vi "Measurement_trial.vi"(0 "I offset":dbl, 2 "input cluster":T1) -> (3 "VR frequency":dbl, 4 "VL frequency":dbl, 5 "PLL output":cluster{dbl, dbl, dbl, dbl}, 6 "RMS values":dbl[](array[numeric]), 7 "Active Power":dbl, 8 "Total power values":dbl[](array[numeric]))   [LabVIEW 2016]
uses:
  <vilib>/measure/matone.llb/Extract Single Tone Information 1 Chan.vi
  <vilib>/measure/NI_MAPro.lvlib
panel:
  in  "dt":dbl=0.000482253 format="%#_13g"
  in  "Numeric":i32=100
  out "I RMS":dbl
  out "VR RMS":dbl
  out "VL RMS":dbl
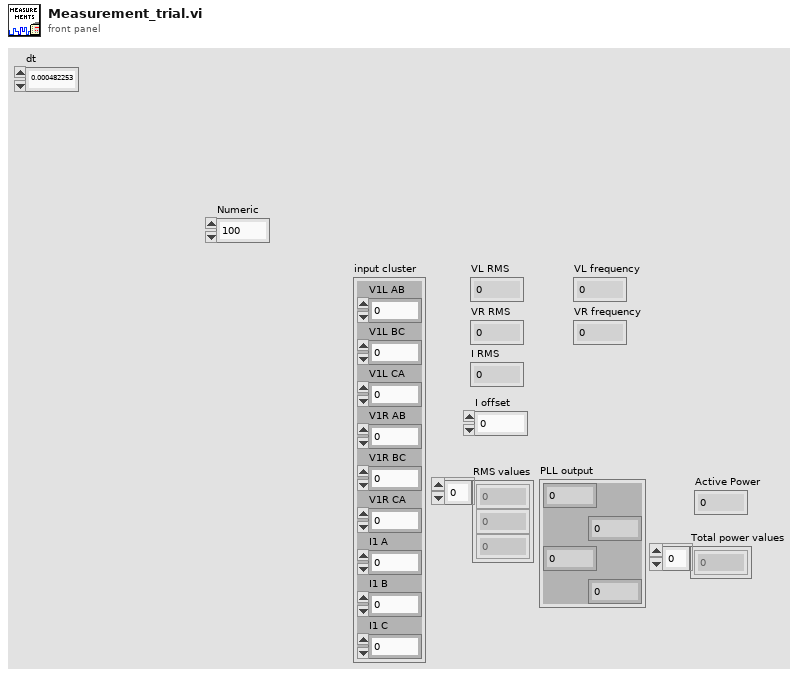
[diagram p1: front panel]
types:
  T1 = cluster{"V1L AB":fxp<+/-,53,11>, "V1L BC":fxp<+/-,53,11>, "V1L CA":fxp<+/-,53,11>, "V1R AB":fxp<+/-,53,11>, "V1R BC":fxp<+/-,53,11>, "V1R CA":fxp<+/-,53,11>, "I1 A":fxp<+/-,53,11>, "I1 B":fxp<+/-,53,11>, "I1 C":fxp<+/-,53,11>}
  T2 = cluster{"V1L AB":fxp<+/-,53,11>, "V1L BC":fxp<+/-,53,11>, "V1L CA":fxp<+/-,53,11>}
  T3 = cluster{"V1R AB":fxp<+/-,53,11>, "V1R BC":fxp<+/-,53,11>, "V1R CA":fxp<+/-,53,11>}
  T4 = cluster{"I1 A":fxp<+/-,53,11>, "I1 B":fxp<+/-,53,11>, "I1 C":fxp<+/-,53,11>}
  T5 = cluster{"t":dbl, "detected phase (deg)":dbl, "detected frequency":dbl, "detected phase (deg)":dbl}
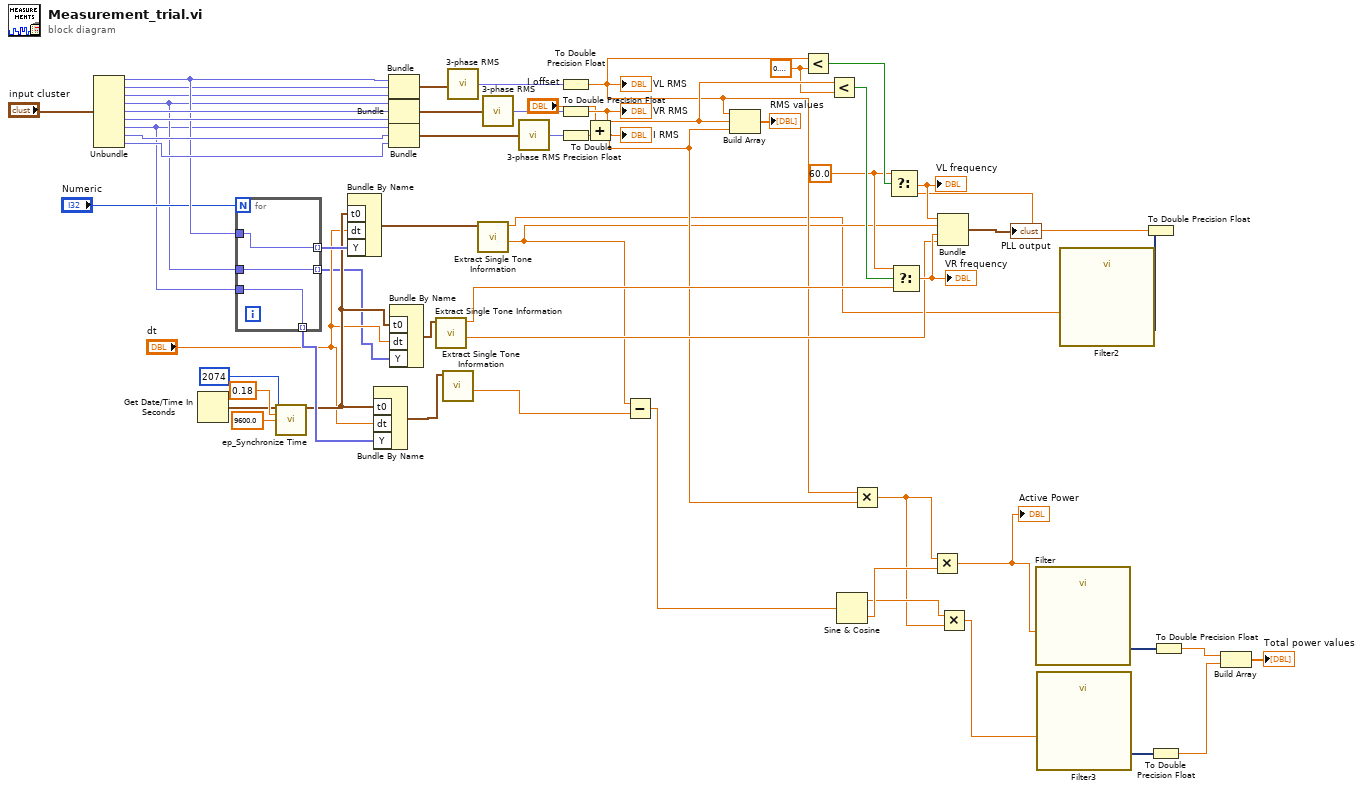
[diagram p0: block diagram]
diagram:
  w48 = 60.0 ("t")
  w51 = 0.30000001192092896 ("y")
  n1 = Unbundle("input cluster") -> ("V1L AB"=w34:fxp<+/-,53,11>, "V1L BC"=w15:fxp<+/-,53,11>, "V1L CA"=w14:fxp<+/-,53,11>, "V1R AB"=w10:fxp<+/-,53,11>, "V1R BC"=w36:fxp<+/-,53,11>, "V1R CA"=w35:fxp<+/-,53,11>, "I1 A"=w9:fxp<+/-,53,11>, "I1 B"=w45:fxp<+/-,53,11>, "I1 C"=w44:fxp<+/-,53,11>)
  n2 = Get Date/Time In Seconds() -> (seconds since 1Jan1904=w28:timestamp)
  n3 = for {
    N: "Numeric" -> [_]
    tunnel: w34 -> [w63]
    tunnel: w10 -> [w62]
    tunnel: [w63] -> w32 mode=indexing
    tunnel: [w62] -> w5 mode=indexing
    tunnel: w9 -> [w61]
    tunnel: [w61] -> w23 mode=indexing
  }
  n4 = call <vilib>:"ep_Synchronize Time.vi"("RT controler time in"=w28, "maximum time difference (sec)"=0.18, "sampling rate (Hz)"=9600.0, "basic calc. interval (samples)"=2074) -> ("RT controler time out"=w7:timestamp)  [unwired: 11 in]
  n5 = Bundle By Name("t0"=w7, "dt"="dt", "Y"=w32) -> (w8:waveform(dbl))  [unwired: 1 in]
  n6 = Bundle By Name("t0"=w7, "dt"="dt", "Y"=w23) -> (w13:waveform(dbl))  [unwired: 1 in]
  n7 = Bundle("V1L AB"=w34, "V1L BC"=w15, "V1L CA"=w14) -> (w59:T2)  [unwired: 1 in]
  n8 = Bundle("V1R AB"=w10, "V1R BC"=w36, "V1R CA"=w35) -> (w58:T3)  [unwired: 1 in]
  n9 = Bundle("I1 A"=w9, "I1 B"=w45, "I1 C"=w44) -> (w57:T4)  [unwired: 1 in]
  n10 = Bundle By Name("t0"=w7, "dt"="dt", "Y"=w5) -> (w4:waveform(dbl))  [unwired: 1 in]
  n11 = call-poly <vilib>:"Extract Single Tone Information.vi"("time signal in"=w4) -> ("detected phase (deg)"=w26:dbl, "detected frequency"=w27:dbl)  [unwired: 5 in, 4 out]
  n12 = call-poly <vilib>:"Extract Single Tone Information.vi"("time signal in"=w13) -> ("detected phase (deg)"=w21:dbl)  [unwired: 5 in, 5 out]
  n13 = call "3-phase RMS.vi"("Vabc"=w59) -> ("RMS"=w55:fxp<+,55,5>)  [unwired: 4 in]
  n14 = call-poly <vilib>:"Extract Single Tone Information.vi"("time signal in"=w8) -> ("detected phase (deg)"=w22:dbl, "detected frequency"=w3:dbl)  [unwired: 5 in, 4 out]
  n15 = call "3-phase RMS.vi"("Vabc"=w58) -> ("RMS"=w54:fxp<+,55,5>)  [unwired: 4 in]
  n16 = call "3-phase RMS.vi"("Vabc"=w57) -> ("RMS"=w56:fxp<+,55,5>)  [unwired: 4 in]
  n17 = To Double Precision Float(number=w55) -> (double precision float=w25:dbl)
  "VL RMS" <- w25
  n18 = To Double Precision Float(number=w54) -> (double precision float=w53:dbl)
  "VR RMS" <- w53
  n19 = To Double Precision Float(number=w56) -> (double precision float=w52:dbl)
  n20 = Add(x="I offset", y=w52) -> (x+y=w24:dbl)
  "I RMS" <- w24
  n21 = Subtract(x=w22, y=w21) -> (x-y=w20:dbl)
  n22 = Build Array(w25, w53, w24) -> (→"RMS values":dbl[])
  n23 = Less?(x=w25, y=w51) -> (x < y?=w50:bool)
  n24 = Less?(x=w53, y=w51) -> (x < y?=w49:bool)
  n25 = Sine & Cosine(0:w20) -> (1:w18:dbl, 2:w19:dbl)
  n26 = Multiply(x=w25, y=w24) -> (x*y=w17:dbl)
  n27 = Select(t=w48, s=w49, f=w27) -> (s? t:f=w46:dbl)
  "VR frequency" <- w46
  n28 = Multiply(x=w17, y=w19) -> (x*y=w12:dbl)
  "Active Power" <- w12
  n29 = Multiply(x=w18, y=w17) -> (x*y=w11:dbl)
  n30 = call "Filter"("Signal"=w12) -> ("Filtered Signal"=w42:dynamicdata)  [unwired: 9 in, 1 out]
  n31 = call "Filter3"("Signal"=w11) -> ("Filtered Signal"=w43:dynamicdata)  [unwired: 9 in, 1 out]
  n32 = call "Filter2"("Signal"=w3) -> ("Filtered Signal"=w2:dynamicdata)  [unwired: 9 in, 1 out]
  n33 = To Double Precision Float(number=w2) -> (double precision float=w1:dbl)
  n34 = Select(t=w48, s=w50, f=w1) -> (s? t:f=w47:dbl)
  "VL frequency" <- w47
  n35 = Bundle("t"=w47, "detected phase (deg)"=w22, "detected frequency"=w46, "detected phase (deg)"=w26) -> (→"PLL output":T5)  [unwired: 1 in]
  n36 = To Double Precision Float(number=w43) -> (double precision float=w40:dbl)
  n37 = To Double Precision Float(number=w42) -> (double precision float=w41:dbl)
  n38 = Build Array(w41, w40) -> (→"Total power values":dbl[])
